vi "Init.vi"(8 "error in (no error)":errorcluster, 11 "XNET Base CFG in":refnum<class "XNET Base CFG.lvclass">) -> (0 "error out":errorcluster, 3 "XNET Base CFG out":refnum<class "XNET Base CFG.lvclass">)   [LabVIEW 2023, in "XNET Base CFG.lvclass"]
uses:
  XNET Base CFG.lvclass
  <vilib>/Utility/error.llb/Error Cluster From Error Code.vi
  <vilib>/ErrorRing/Error Ring.xnode
  XNET Base CFG.lvclass/XNET Base CFG.ctl
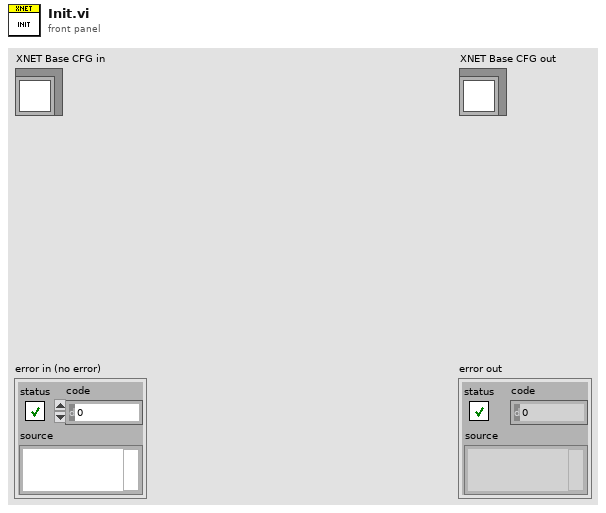
[diagram p1: front panel]
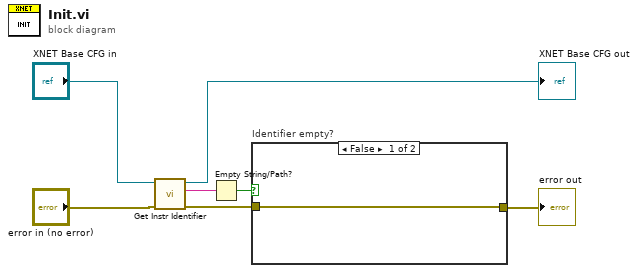
[diagram p0: block diagram]
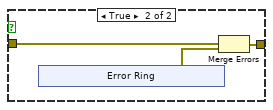
[diagram p2: hidden frame]
diagram:
  n1 = call-dynamic "Get Instr Identifier.vi"("error in (no error)"="error in (no error)", "Configuration Base in"="XNET Base CFG in") -> ("error out"=w7:errorcluster, "Instr Identifier"=w5:string, "Configuration Base out"=→"XNET Base CFG out":refnum<class "XNET Base CFG.lvclass">)  [unwired: 7 in]
  n2 = Empty String/Path?(string/path=w5) -> (empty?=w6:bool)
  n3 = case "Identifier empty?" shown="False" w6 {
    tunnel: w7 -> [w8 w11]
    tunnel: [w8 w10] -> w1
    frame False {
    }
    frame True {
      n4 = xnode "Error Ring"() -> ("error out"=w9:errorcluster)
      n5 = Merge Errors(w11, w9) -> (w10:errorcluster)
    }
  }
  "error out" <- w1
